vi "get_settings_cluster.vi"(8 "error in (no error)":errorcluster, 11 "GenericPlugin in":refnum<class "TrajectoryMG100122AODFrameScan.lvclass">) -> (0 "error out":errorcluster, 2 "settings cluster":variant, 3 "GenericPlugin out":refnum<class "TrajectoryMG100122AODFrameScan.lvclass">)   [LabVIEW 2010, in "TrajectoryMG100122AODFrameScan.lvclass"]
uses:
  TrajectoryMG100122AODFrameScan.lvclass
  TrajectoryMG100122AODFrameScan.lvclass/TrajectoryMG100122AODFrameScan.ctl
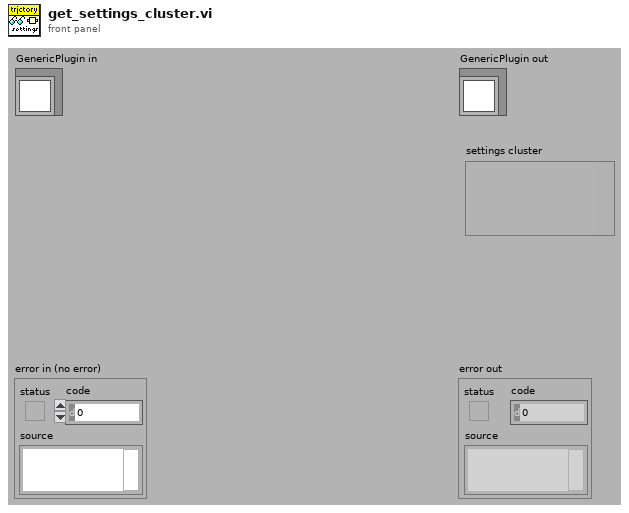
[diagram p1: front panel]
types:
  T1 = typedef "TrajectoryMG100122AODFrameScan.lvclass/settings_cluster.ctl" = cluster{"x resolution":i32, "y resolution":i32, "pixel dwell time":dbl[unit], "transformation factors":dbl[unit][], "ratio factors x":dbl, "ratio factors y":dbl}
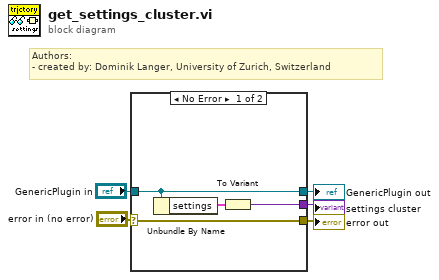
[diagram p0: block diagram]
diagram:
  # "Authors: \n- created by: Dominik Langer, University of Zurich, Switzerland"
  n1 = case shown="No Error" "error in (no error)" {
    selector: "error in (no error)" -> [w7 w10]
    tunnel: "GenericPlugin in" -> [w6 w11]
    tunnel: [w8 _] -> w3
    tunnel: [w7 w10] -> w2
    tunnel: [w6 w11] -> w1
    frame No Error {
      n2 = Unbundle By Name(w6) -> ("settings"=w9:T1)
      n3 = To Variant(anything=w9) -> (Variant=w8:variant)
    }
    frame Error {
    }
  }
  "error out" <- w2
  "GenericPlugin out" <- w1
  "settings cluster" <- w3
